vi "CgRawInterp.vi"(2 "Time Bytes Before Output":i16, 3 "Cyberglove Out":string) -> (0 "Raw Data":u8[](array[numeric]), 1 "Time":i32)   [LabVIEW 2012]
doc: "Grabs the byte stream from the cyberglove data collect program, removes the time bytes, and then processes each byte as a number between 1-255 to create an array of raw data for each of the sensors."
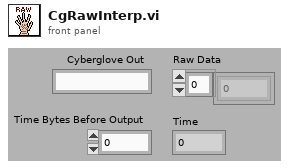
[diagram p1: front panel]
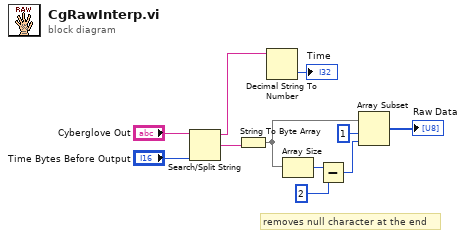
[diagram p0: block diagram]
diagram:
  # "removes null character at the end"
  n1 = Search/Split String(string="Cyberglove Out", offset (0)="Time Bytes Before Output") -> (substring before match=w3:string, match + rest of string=w4:string)  [unwired: 1 in, 1 out]
  n2 = String To Byte Array(string=w4) -> (unsigned byte array=w11:u8[])
  n3 = Decimal String To Number(string=w3) -> (number=→"Time":i32)  [unwired: 2 in, 1 out]
  n4 = Array Size(array=w11) -> (size(s)=w9:i32)
  n5 = Subtract(x=w9, y=2) -> (x-y=w7:i32)
  n6 = Array Subset(array=w11, index=1, length=w7) -> (→"Raw Data":u8[])
